vi "quoridor_server.vi"() -> ()   [LabVIEW 2015]
panel:
  in  "STOP":bool
  in  "NON":bool
  in  "OUI":bool
  out "String 6":string
  out "String 5":string
  out "String 4":string
  out "String 3":string
  out "LED1":bool
  out "LED2":bool
  out "LED3":bool
  out "String 2":string
  out "String":string
  out "Play Led":bool
  out "Victoire Client":bool
  out "Victoire Joueur Serveur":bool
  out "?":string
  out "Nombre de murs restants":i32
  out "Timeout":dbl
  out "COMPTEUR LED":dbl
  out "Etat jeu":string
  out "Position joueur":dbl[](array[numeric])
  in  "Bouton gauche (8)":bool
  in  "Bouton droite (4)":bool
  in  "Bouton bas (1)":bool
  in  "Bouton haut (2)":bool
  in  "passer tour":bool
  in  "Haut":bool
  in  "Droite":bool
  in  "X":i32(slide) scale=0.0..8.0
  in  "Y":i32(slide)
  out "Array":u32[][](array[ring])
  # "Règles du jeu : Inspiration Quoridor  \n\nLe but est d’atteindre la ligne d’arrivée à l’autre bout du plateau, rien de plus simple ! \n\nPour cela le joueur peut se déplacer, ou alors poser un mur pour entraver l’adversaire. \n\nLes murs font 2 cases de long, on peut les placer Verticaux ou Horizontaux en sélectionnant la case avec les deux curseurs. \n\nLors des déplacements, un joueur ne peut pas franchir un mur, ni sortir du plateau et encore moins marcher sur l’adversaire ! \n\nEt voilà qui conclut cette explication, bonne chance joueur !"
  # "PS : Ne pas enfermer l’adversaire ni bloquer tous les chemins possibles svp au risque de casser le fun…"
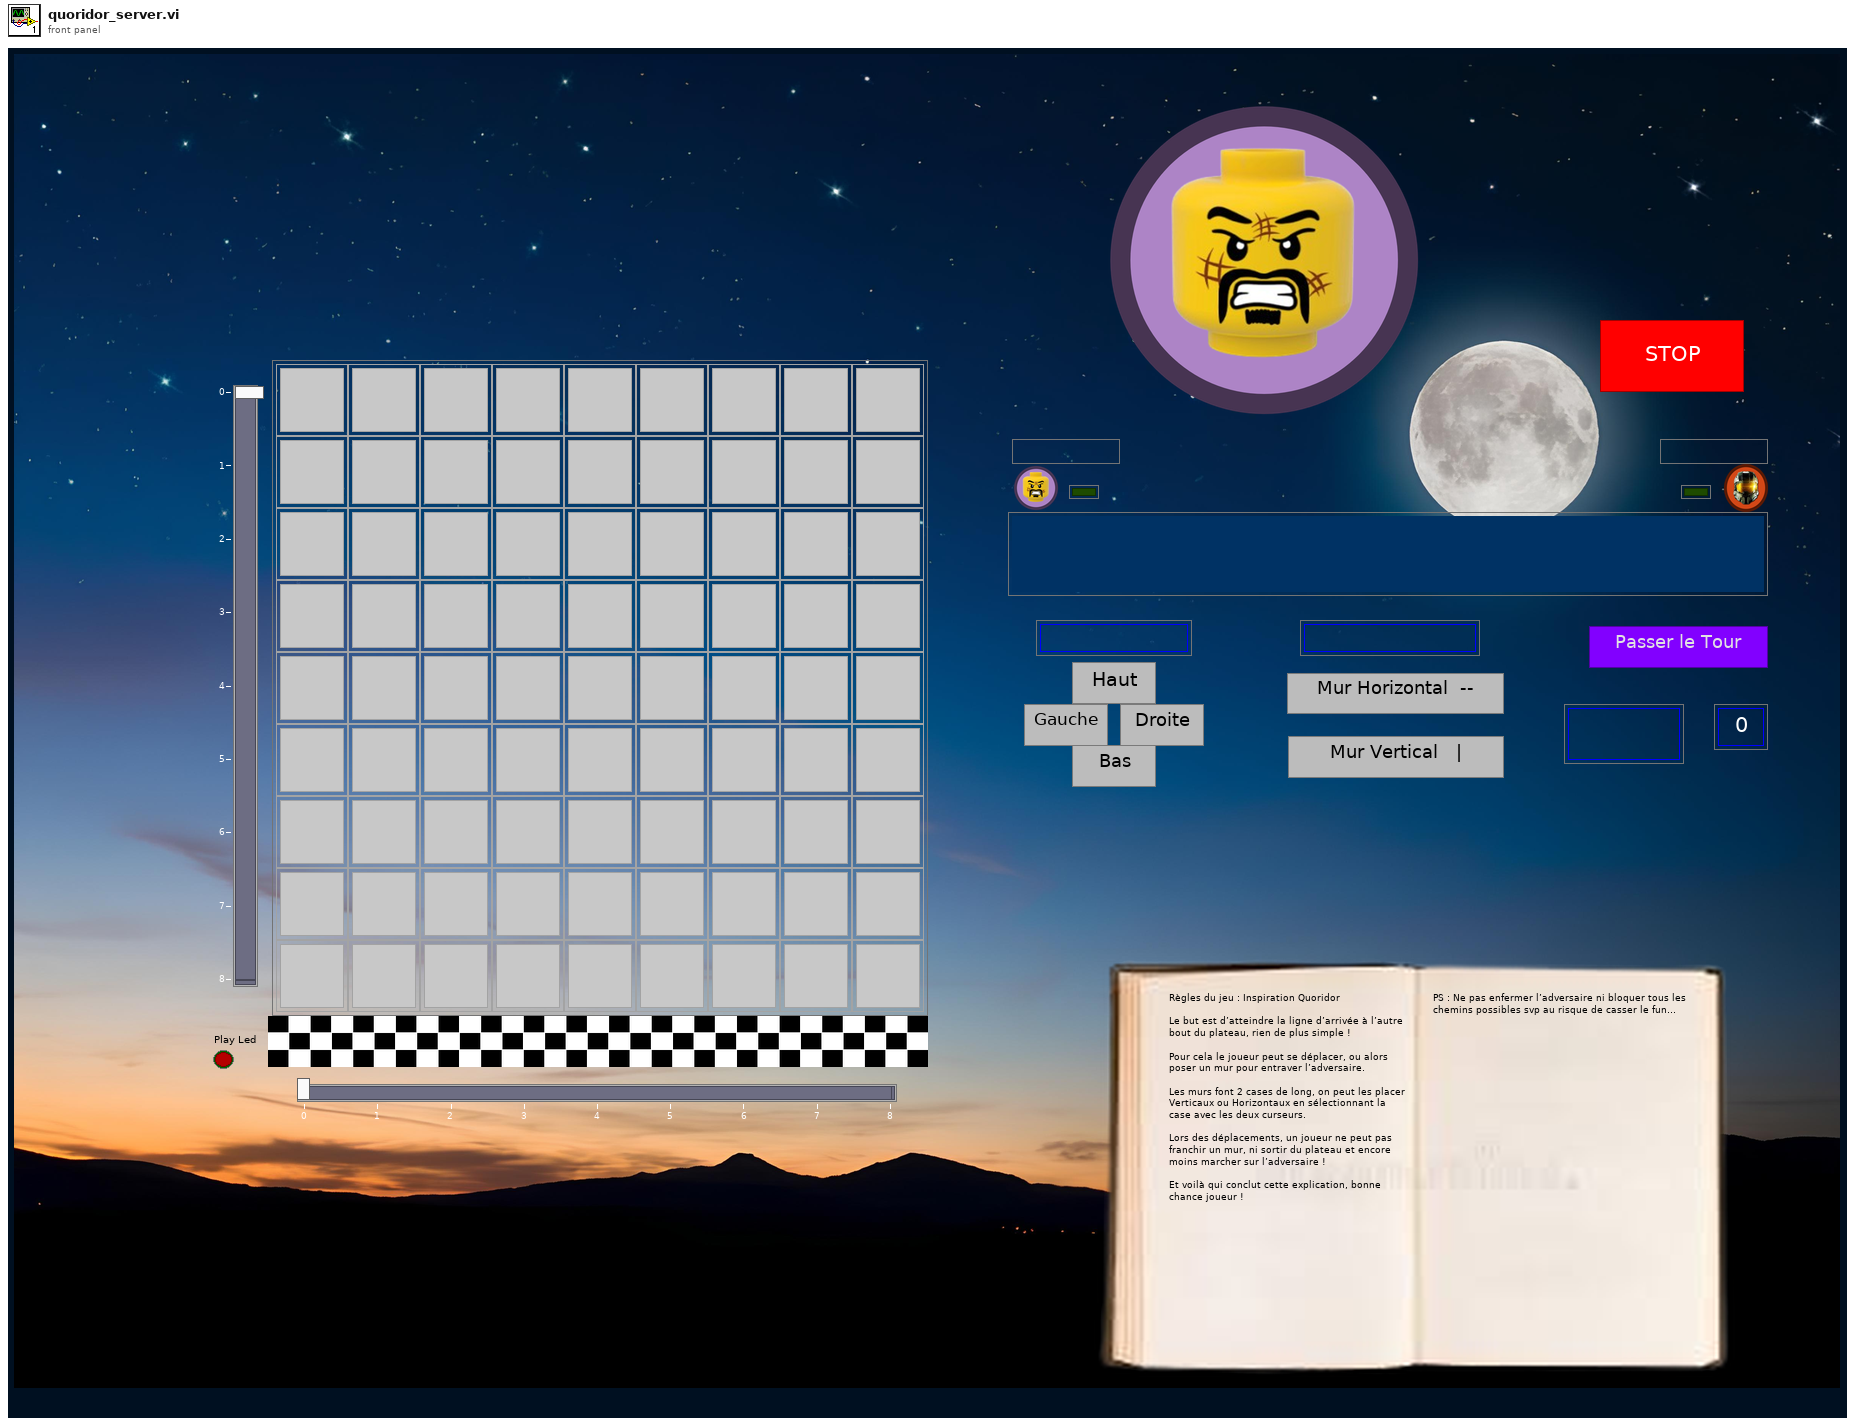
[diagram p1: front panel]
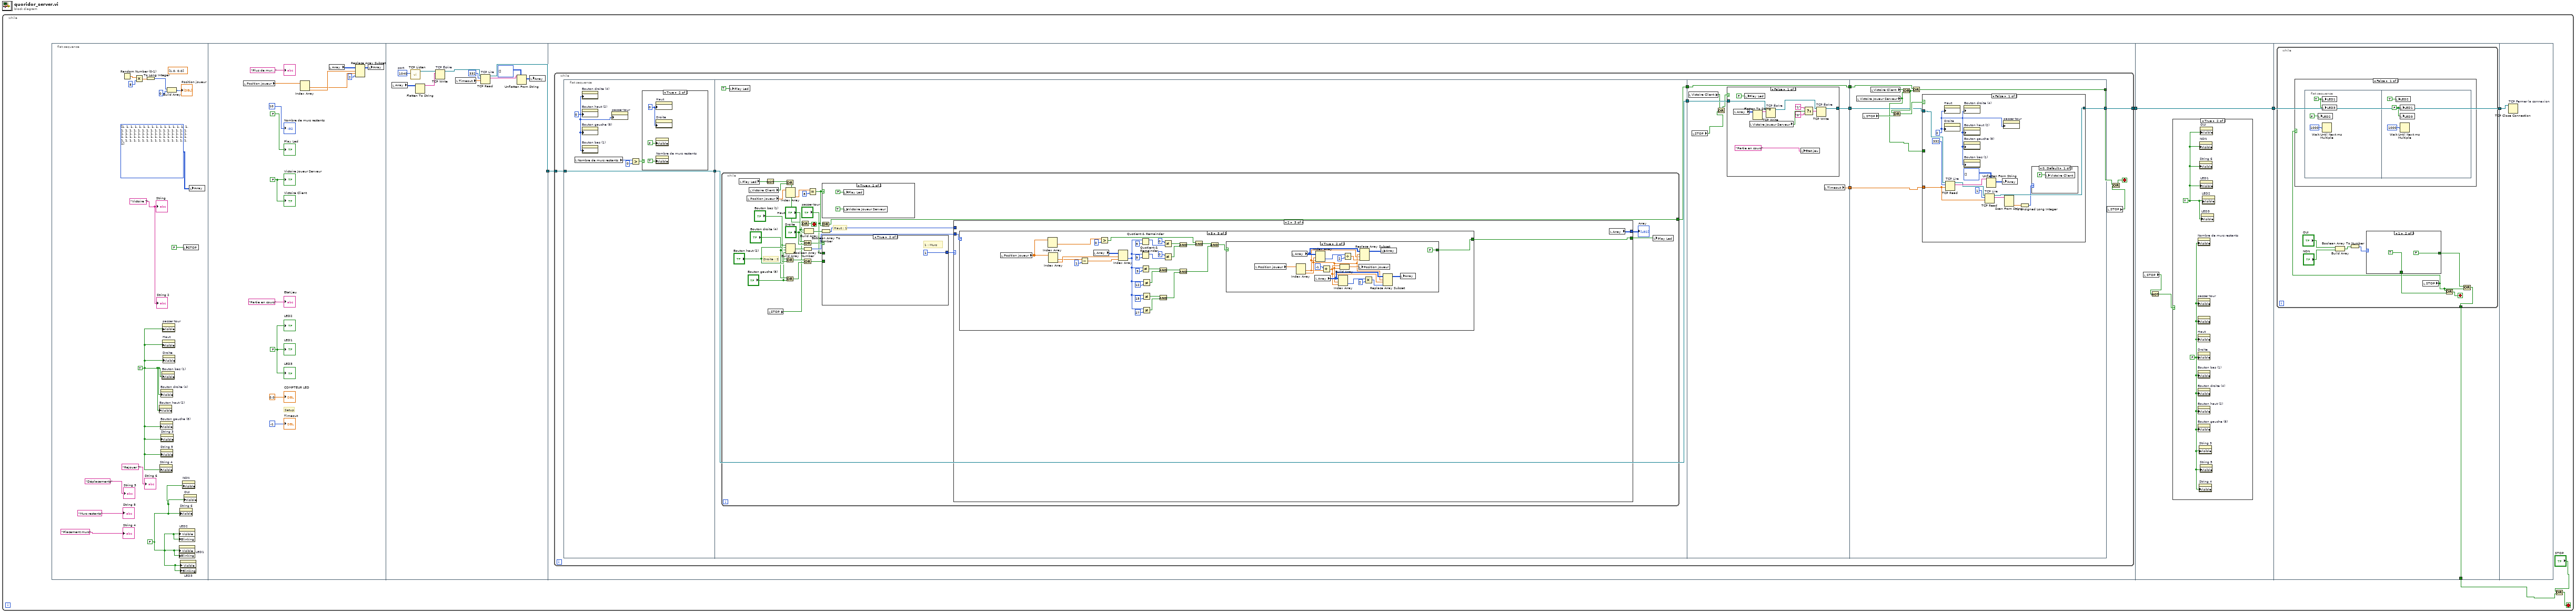
[diagram p0: block diagram]
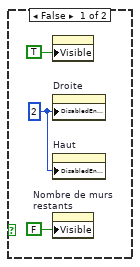
[diagram p2: hidden frame]
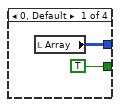
[diagram p4: hidden frame]
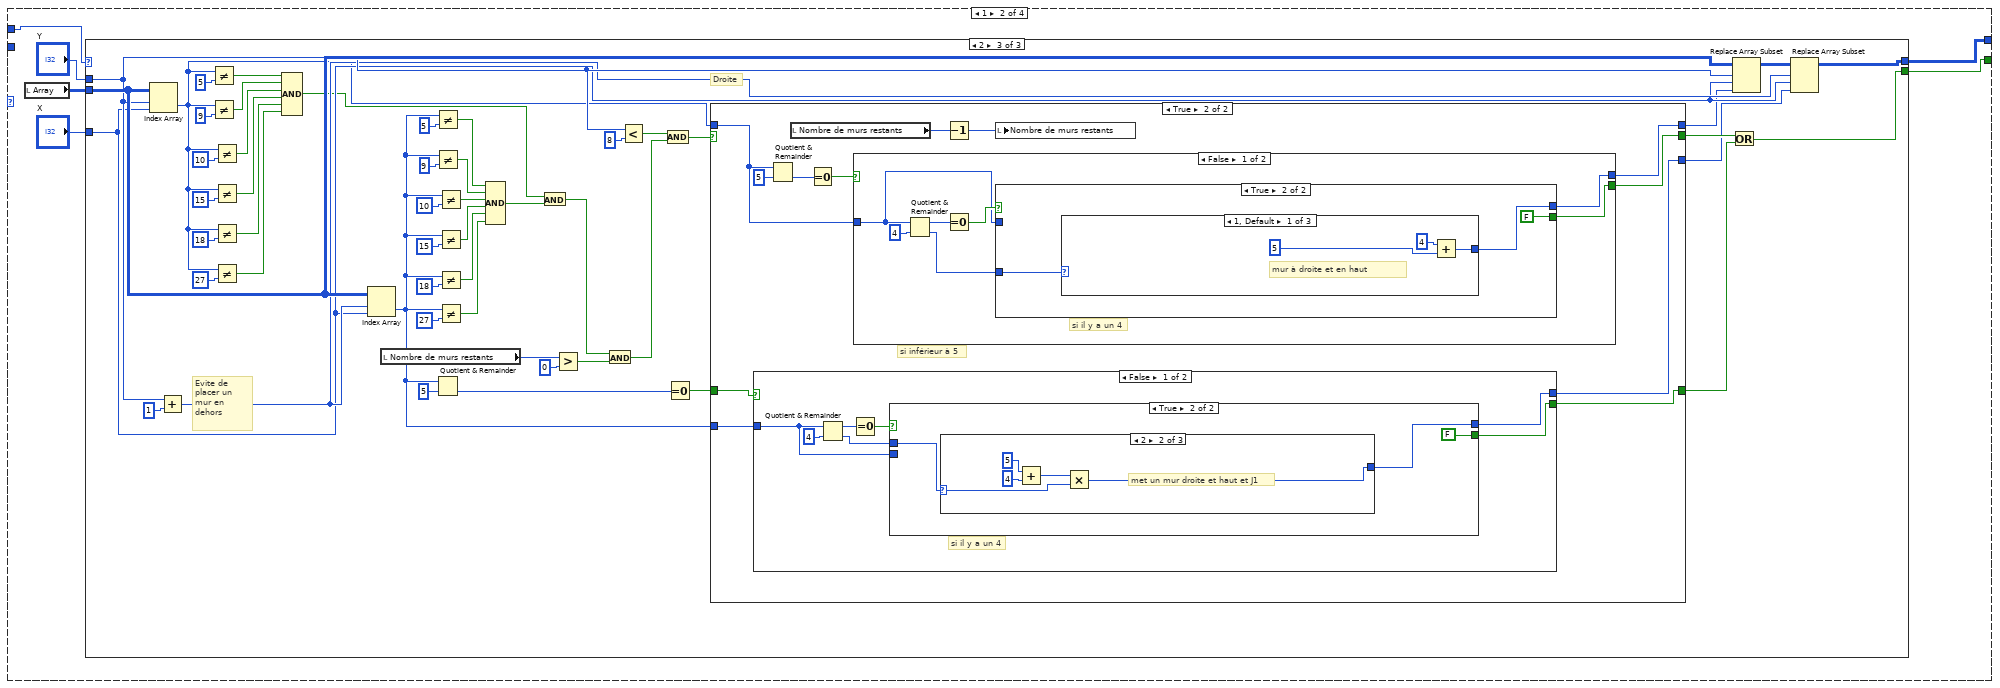
[diagram p5: hidden frame]
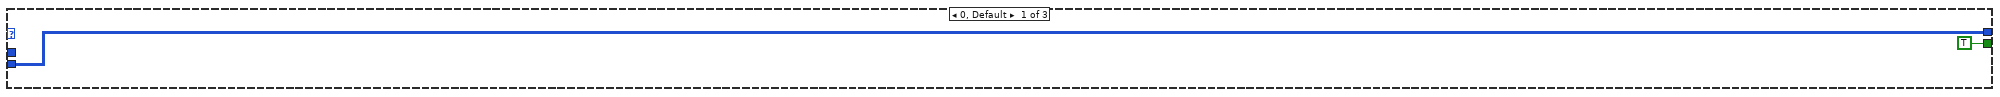
[diagram p6: hidden frame]
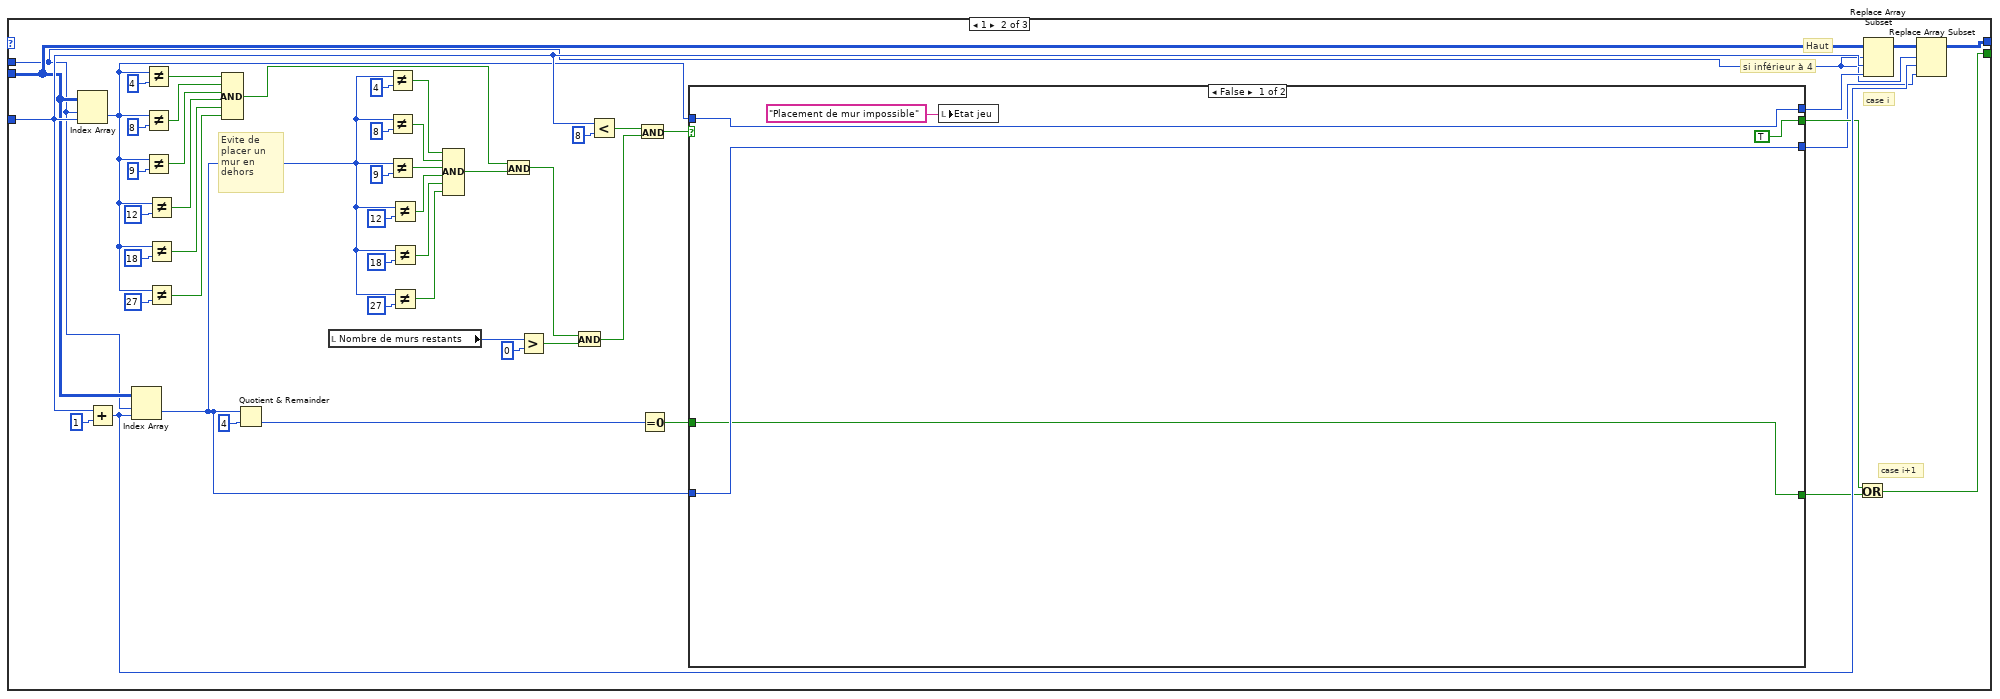
[diagram p7: hidden frame]
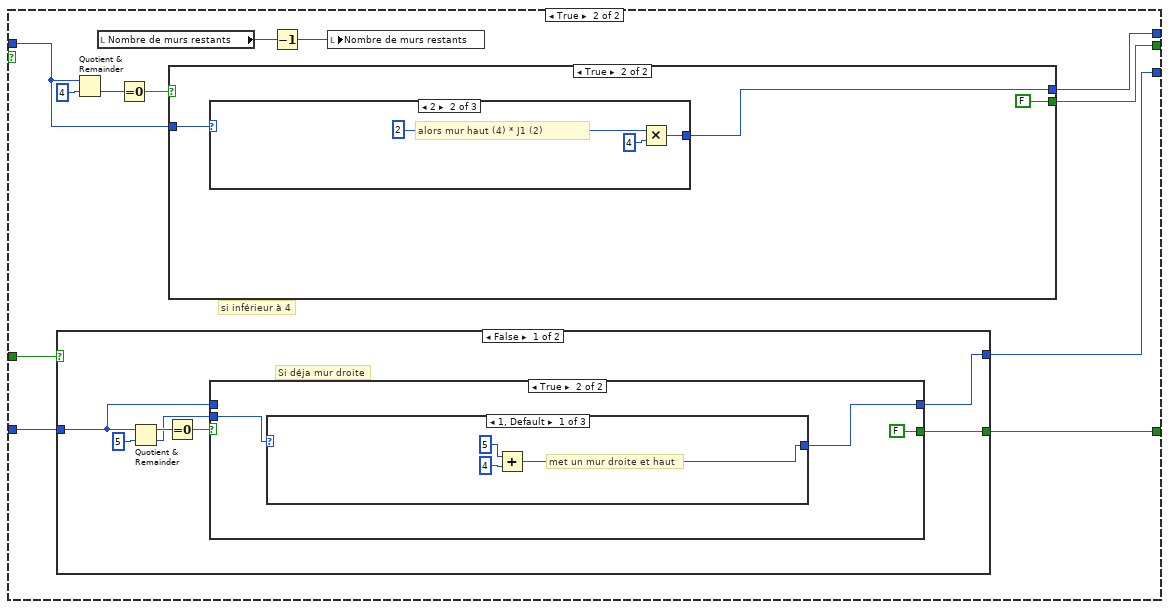
[diagram p8: hidden frame]
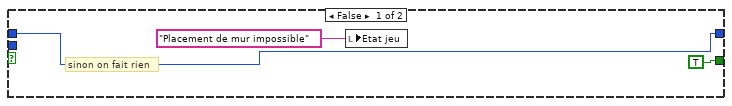
[diagram p9: hidden frame]
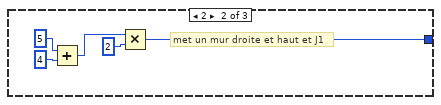
[diagram p10: hidden frame]
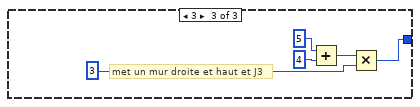
[diagram p11: hidden frame]
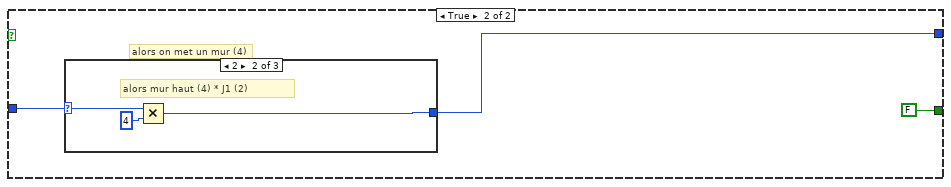
[diagram p12: hidden frame]
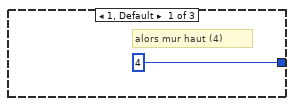
[diagram p13: hidden frame]
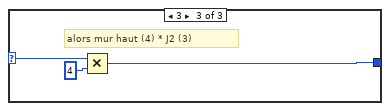
[diagram p14: hidden frame]
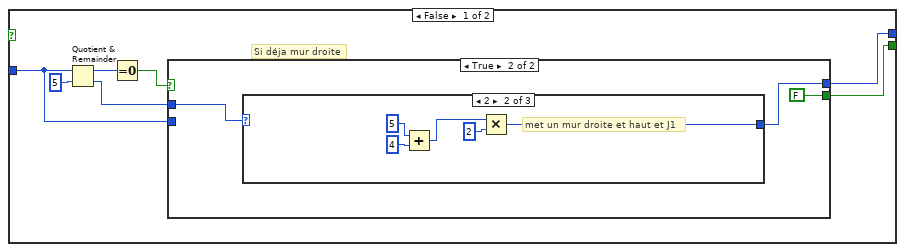
[diagram p15: hidden frame]
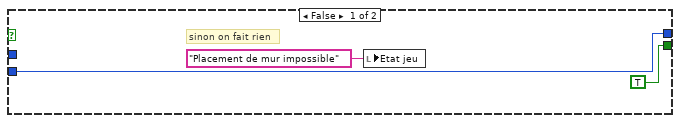
[diagram p16: hidden frame]
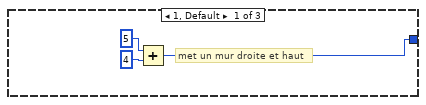
[diagram p17: hidden frame]
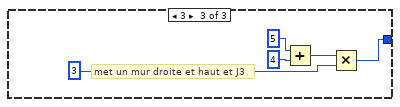
[diagram p18: hidden frame]
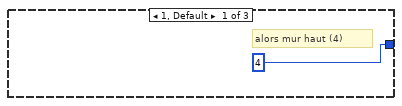
[diagram p19: hidden frame]
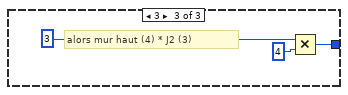
[diagram p20: hidden frame]
diagram:
  n1 = while {
    stop <- w3 stop-if-true
    n2 = flat-sequence {
      tunnel: [w39] -> w7
      tunnel: w7 -> [w48]
      tunnel: [w49] -> w6
      tunnel: w6 -> [w678]
      tunnel: [w678] -> w5
      tunnel: w5 -> [w682]
      tunnel: [w682] -> w4
      tunnel: [w681] -> w1
      tunnel: w4 -> [w703]
      frame #0 {
        w13 = FALSE
        w14 = TRUE
        w15 = "Victoire ?"
        (unwired) dbl[] [1.0, 0.0] ("Position joueur")
        n3 = Random Number (0-1)() -> (number: 0 to 1=w20:dbl)
        n4 = Multiply(x=w20, y=8) -> (x*y=w22:dbl)
        n5 = To Long Integer(number=w22) -> (32bit integer=w17:i32)
        n6 = property on="Bouton haut (2)" class="Bool"("Visible"=w14) -> ()  [unwired: 2 in, 2 out]
        n7 = property on="String 4" class="Str"("Visible"=w14) -> ()  [unwired: 2 in, 2 out]
        n8 = property on="Bouton gauche (8)" class="Bool"("Visible"=w14) -> ()  [unwired: 2 in, 2 out]
        n9 = property on="Bouton droite (4)" class="Bool"("Visible"=w14) -> ()  [unwired: 2 in, 2 out]
        n10 = property on="String 5" class="Str"("Visible"=w14) -> ()  [unwired: 2 in, 2 out]
        n11 = property on="String 3" class="Str"("Visible"=w14) -> ()  [unwired: 2 in, 2 out]
        n12 = property on="Bouton bas (1)" class="Bool"("Visible"=w14) -> ()  [unwired: 2 in, 2 out]
        n13 = property on="passer tour" class="Bool"("Visible"=w14) -> ()  [unwired: 2 in, 2 out]
        n14 = property on="Haut" class="Bool"("Visible"=w14) -> ()  [unwired: 2 in, 2 out]
        n15 = property on="Droite" class="Bool"("Visible"=w14) -> ()  [unwired: 2 in, 2 out]
        n16 = Build Array(w17, 0) -> (→"Position joueur":i32[])
        n17 = property on="LED2" class="Bool (strict)"("Visible"=w13, "Blinking"=w13) -> ()  [unwired: 2 in, 2 out]
        n18 = property on="LED1" class="Bool (strict)"("Visible"=w13, "Blinking"=w13) -> ()  [unwired: 2 in, 2 out]
        n19 = property on="String 6" class="Str"("Visible"=w13) -> ()  [unwired: 2 in, 2 out]
        n20 = property on="LED3" class="Bool (strict)"("Visible"=w13, "Blinking"=w13) -> ()  [unwired: 2 in, 2 out]
        n21 = property on="NON" class="Bool"("Visible"=w13) -> ()  [unwired: 2 in, 2 out]
        n22 = local write "STOP"(FALSE) -> ()
        n23 = property on="OUI" class="Bool"("Visible"=w13) -> ()  [unwired: 2 in, 2 out]
        n24 = local write "Array"(i32[][] [[1, 1, 1, 1, 1, 1, 1, 1, 1], [1, 1, 1, 1, 1, 1, 1, 1, 1], [1, 1, 1, 1, 1, 1, 1, 1, 1], [1, 1, 1, 1, 1, 1, 1, 1, 1], [1, 1, 1, 1, 1, 1, 1, 1, 1], [1, 1, 1, 1, 1, 1, 1, 1, 1], [1, 1, 1, 1, 1, 1, 1, 1, 1], [1, 1, 1, 1, 1, 1, 1, 1, 1], [1, 1, 1, 1, 1, 1, 1, 1, 1]] ("Array 2")) -> ()
        "String" <- w15
        "String 2" <- w15
        "String 3" <- "Déplacements"
        "String 5" <- "Murs restants"
        "String 4" <- "Placement murs"
        "String 6" <- "Rejouer ?"
      }
      frame #1 {
        w23 = FALSE
        w34 = FALSE
        # "Setup"
        n25 = local read "Position joueur"() -> (w32:dbl[])
        n26 = Index Array(array=w32) -> (element #1=w28:dbl, element #2=w29:dbl)  [unwired: 2 in]
        n27 = local read "Array"() -> (w30:u32[][])
        n28 = Replace Array Subset(array=w30, new element=2, index (row)=w29, index (col)=w28) -> (w31:u32[][])
        n29 = local write "Array"(w31) -> ()
        "COMPTEUR LED" <- 0.0
        "Etat jeu" <- "Partie en cours"
        "LED3" <- w34
        "LED1" <- w34
        "LED2" <- w34
        "Timeout" <- -1
        "Play Led" <- FALSE
        "Nombre de murs restants" <- 10
        "?" <- "Plus de mur..."
        "Victoire Joueur Serveur" <- w23
        "Victoire Client" <- w23
      }
      frame #2 {
        w44 = u16 1040  # port
        n30 = local read "Array"() -> (w46:u32[][])
        n31 = call <vilib>:"TCP Listen.vi"("port"=w44) -> ("connection ID"=w47:refnum<k5>)  [unwired: 6 in, 4 out]
        n32 = Flatten To String(anything=w46) -> (data string=w45:string)  [unwired: 3 in, 2 out]
        n33 = TCP Write "TCP Écrire"(connection ID=w47, data in=w45) -> (connection ID out=w40:refnum<k5>)  [unwired: 2 in, 2 out]
        n34 = local read "Timeout"() -> (w38:dbl)
        n35 = TCP Read "TCP Lire"(connection ID=w40, bytes to read=332, 9:w38) -> (connection ID out=w39:refnum<k5>, data out=w42:string)  [unwired: 2 in, 1 out]
        n36 = Unflatten From String(type=i32[][] [], binary string=w42) -> (value=w37:i32[][])  [unwired: 3 in, 2 out]
        n37 = local write "Array"(w37) -> ()
      }
      frame #3 {
        n38 = while {
          tunnel: [w60] -> w49
          tunnel: w48 -> [w58]
          stop <- w51 stop-if-true
          n39 = flat-sequence {
            tunnel: w58 -> [w65]
            tunnel: [w65] -> w54
            tunnel: [w74] -> w57
            tunnel: [w72] -> w55
            tunnel: w54 -> [w74]
            tunnel: [w629] -> w59
            tunnel: w57 -> [w631]
            tunnel: [w630] -> w56
            tunnel: w55 -> [w628]
            tunnel: [w628] -> w53
            tunnel: [w649] -> w60
            tunnel: w59 -> [w646]
            tunnel: w56 -> [w645]
            tunnel: w53 -> [w653]
            tunnel: [w652] -> w52
            frame #0 {
              w61 = 0
              n40 = local read "Nombre de murs restants"() -> (w62:i32)
              n41 = property on="Bouton droite (4)" class="Bool"("DisabledEnum"=w61) -> ()  [unwired: 2 in, 2 out]
              n42 = property on="Bouton haut (2)" class="Bool"("DisabledEnum"=w61) -> ()  [unwired: 2 in, 2 out]
              n43 = property on="Bouton gauche (8)" class="Bool"("DisabledEnum"=w61) -> ()  [unwired: 2 in, 2 out]
              n44 = property on="Bouton bas (1)" class="Bool"("DisabledEnum"=w61) -> ()  [unwired: 2 in, 2 out]
              n45 = property on="passer tour" class="Bool"("DisabledEnum"=w61) -> ()  [unwired: 2 in, 2 out]
              n46 = Greater?(x=w62, y=0) -> (0:w63:bool)
              n47 = case shown="True" w63 {
                frame False {
                  w68 = 2
                  n48 = property class="Str"("Visible"=TRUE) -> ()  [unwired: 2 in, 2 out]
                  n49 = property on="Droite" class="Bool"("DisabledEnum"=w68) -> ()  [unwired: 2 in, 2 out]
                  n50 = property on="Haut" class="Bool"("DisabledEnum"=w68) -> ()  [unwired: 2 in, 2 out]
                  n51 = property on="Nombre de murs restants" class="DigNum (strict)"("Visible"=FALSE) -> ()  [unwired: 2 in, 2 out]
                }
                frame True {
                  w71 = 0
                  n52 = property on="Haut" class="Bool"("DisabledEnum"=w71) -> ()  [unwired: 2 in, 2 out]
                  n53 = property on="Droite" class="Bool"("DisabledEnum"=w71) -> ()  [unwired: 2 in, 2 out]
                  n54 = property class="Str"("Visible"=FALSE) -> ()  [unwired: 2 in, 2 out]
                  n55 = property on="Nombre de murs restants" class="DigNum (strict)"("Visible"=TRUE) -> ()  [unwired: 2 in, 2 out]
                }
              }
            }
            frame #1 {
              n56 = while {
                tunnel: [w78] -> w72
                stop <- w76 stop-if-true
                # "Haut : 1"
                # "Droite : 2"
                n57 = local read "Play Led"() -> (w93:bool)
                n58 = local read "Position joueur"() -> (w81:dbl[])
                n59 = local read "Victoire Client"() -> (w84:bool)
                n60 = Not(x=w93) -> (.not. x?=w85:bool)
                n61 = local read "STOP"() -> (w75:bool)
                n62 = Or(x=w85, y=w84) -> (x .or. y?=w77:bool)
                n63 = Or(x="Bouton haut (2)", y="Bouton bas (1)") -> (x .or. y?=w98:bool)
                n64 = Or(x="Bouton droite (4)", y="Bouton gauche (8)") -> (x .or. y?=w99:bool)
                n65 = Index Array(array=w81) -> (element #2=w82:dbl)  [unwired: 2 in, 1 out]
                n66 = Build Array("Bouton bas (1)", "Bouton haut (2)", "Bouton droite (4)", "Bouton gauche (8)") -> (w100:bool[])
                n67 = Or(x=w77, y=w75) -> (x .or. y?=w76:bool)
                n68 = Or(x="Haut", y="Droite") -> (x .or. y?=w92:bool)
                n69 = Or(x=w98, y=w99) -> (x .or. y?=w91:bool)
                n70 = Boolean Array To Number(Boolean array=w100) -> (number=w88:u32)
                n71 = Build Array("Haut", "Droite") -> (w103:bool[])
                n72 = Equal?(x=w82, y=8) -> (x = y?=w80:bool)
                n73 = Or(x="passer tour", y=w80) -> (x .or. y?=w78:bool)
                n74 = Boolean Array To Number(Boolean array=w103) -> (number=w89:u32)
                n75 = case shown="True" w80 {
                  frame False {
                  }
                  frame True {
                    n76 = local write "Play Led"(FALSE) -> ()
                    n77 = local write "Victoire Joueur Serveur"(TRUE) -> ()
                  }
                }
                n78 = case shown="True" w92 {
                  tunnel: [w618 1] -> w90
                  tunnel: "passer tour" -> [w617 _]
                  tunnel: w91 -> [w616 _]
                  frame False {
                    n79 = case shown="False" w616 {
                      tunnel: [w620 2] -> w618
                      tunnel: w617 -> [w619 _]
                      frame False {
                        n80 = case shown="False" w619 {
                          tunnel: [0 3] -> w620
                          frame False {
                            # "0"
                          }
                          frame True {
                            # "3 : Abandon"
                          }
                        }
                      }
                      frame True {
                        # "2 : Pion"
                      }
                    }
                  }
                  frame True {
                    # "1 : Murs"
                  }
                }
                n81 = case shown="2" w90 {
                  tunnel: w89 -> [_ w112 _ _]
                  tunnel: [w107 w109 w399 w615] -> w86
                  tunnel: w88 -> [_ _ w401 _]
                  tunnel: [TRUE w108 w400 FALSE] -> w87
                  frame 0, Default {
                    n82 = local read "Array"() -> (w107:u32[][])
                  }
                  frame 1 {
                    n83 = local read "Array"() -> (w113:u32[][])
                    n84 = case shown="2" w112 {
                      tunnel: w113 -> [w115 w161 w301]
                      tunnel: "Y" -> [_ w159 w300]
                      tunnel: "X" -> [_ w162 w298]
                      tunnel: [w115 w156 w296] -> w109
                      tunnel: [TRUE w155 w295] -> w108
                      frame 0, Default {
                      }
                      frame 1 {
                        # "si inférieur à 4"
                        # "case i+1"
                        # "case i"
                        # "Evite de placer un mur en dehors"
                        # "Haut"
                        n85 = Index Array(array=w161, index (row)=w159, index (col)=w162) -> (element=w122:u32)
                        n86 = Add(x=w162, y=1) -> (x+y=w160:i32)
                        n87 = Index Array(array=w161, index (row)=w159, index (col)=w160) -> (element=w123:u32)
                        n88 = Not Equal?(x=w122, y=4) -> (x != y?=w144:bool)
                        n89 = Not Equal?(x=w122, y=8) -> (x != y?=w143:bool)
                        n90 = Not Equal?(x=w122, y=9) -> (x != y?=w142:bool)
                        n91 = Not Equal?(x=w122, y=12) -> (x != y?=w141:bool)
                        n92 = Not Equal?(x=w122, y=18) -> (x != y?=w140:bool)
                        n93 = Not Equal?(x=w122, y=27) -> (x != y?=w139:bool)
                        n94 = Compound Arithmetic op=AND(w144, w143, w142, w141, w140, w139) -> (w127:bool)
                        n95 = Quotient & Remainder(x=w123, y=4) -> (floor(x/y)=w157:u32)  [unwired: 1 out]
                        n96 = local read "Nombre de murs restants"() -> (w119:i32)
                        n97 = Not Equal?(x=w123, y=4) -> (x != y?=w133:bool)
                        n98 = Not Equal?(x=w123, y=8) -> (x != y?=w132:bool)
                        n99 = Not Equal?(x=w123, y=9) -> (x != y?=w131:bool)
                        n100 = Not Equal?(x=w123, y=12) -> (x != y?=w130:bool)
                        n101 = Not Equal?(x=w123, y=18) -> (x != y?=w129:bool)
                        n102 = Not Equal?(x=w123, y=27) -> (x != y?=w128:bool)
                        n103 = Compound Arithmetic op=AND(w133, w132, w131, w130, w129, w128) -> (w126:bool)
                        n104 = And(x=w127, y=w126) -> (x .and. y?=w118:bool)
                        n105 = Greater?(x=w119, y=0) -> (0:w116:bool)
                        n106 = And(x=w118, y=w116) -> (x .and. y?=w117:bool)
                        n107 = Less?(x=w162, y=8) -> (x < y?=w124:bool)
                        n108 = And(x=w124, y=w117) -> (x .and. y?=w125:bool)
                        n109 = Equal To 0?(x=w157) -> (x = 0?=w153:bool)
                        n110 = case shown="False" w125 {
                          tunnel: [w171 w180] -> w164
                          tunnel: w122 -> [w171 w179]
                          tunnel: [TRUE w178] -> w154
                          tunnel: w153 -> [w168 w177]
                          tunnel: w123 -> [w169 w176]
                          tunnel: [w168 w175] -> w152
                          tunnel: [w169 w174] -> w151
                          frame False {
                            n111 = local write "Etat jeu"("Placement de mur impossible") -> ()
                          }
                          frame True {
                            # "si inférieur à 4"
                            n112 = case shown="False" w177 {
                              tunnel: [w187 w212] -> w174
                              tunnel: w176 -> [w185 w211]
                              tunnel: [w184 FALSE] -> w175
                              frame False {
                                # "Si déja mur droite"
                                n113 = Quotient & Remainder(x=w185, y=5) -> (x-y*floor(x/y)=w188:u32, floor(x/y)=w186:u32)
                                n114 = Equal To 0?(x=w188) -> (x = 0?=w189:bool)
                                n115 = case shown="True" w189 {
                                tunnel: w186 -> [_ w196]
                                tunnel: [w193 w195] -> w187
                                tunnel: w185 -> [w193 _]
                                tunnel: [TRUE FALSE] -> w184
                                frame False {
                                # "sinon on fait rien"
                                n116 = local write "Etat jeu"("Placement de mur impossible") -> ()
                                }
                                frame True {
                                n117 = case shown="1, Default" w196 {
                                tunnel: [w198 w201 w206] -> w195
                                frame 1, Default {
                                # "met un mur droite et haut"
                                n118 = Add(x=5, y=4) -> (x+y=w198:i32)
                                }
                                frame 2 {
                                # "met un mur droite et haut et J1"
                                n119 = Add(x=5, y=4) -> (x+y=w202:i32)
                                n120 = Multiply(x=w202, y=2) -> (x*y=w201:i32)
                                }
                                frame 3 {
                                # "met un mur droite et haut et J3"
                                n121 = Add(x=5, y=4) -> (x+y=w207:i32)
                                n122 = Multiply(x=w207, y=3) -> (x*y=w206:i32)
                                }
                                }
                                }
                                }
                              }
                              frame True {
                                # "alors on met un mur (4)"
                                n123 = case shown="2" w211 {
                                selector: w211 -> [_ w214 w217]
                                tunnel: [4 w215 w218] -> w212
                                frame 1, Default {
                                # "alors mur haut (4)"
                                }
                                frame 2 {
                                # "alors mur haut (4) * J1 (2)"
                                n124 = Multiply(x=w214, y=4) -> (x*y=w215:u32)
                                }
                                frame 3 {
                                # "alors mur haut (4) * J2 (3)"
                                n125 = Multiply(x=w217, y=4) -> (x*y=w218:u32)
                                }
                                }
                              }
                            }
                            n126 = Quotient & Remainder(x=w179, y=4) -> (floor(x/y)=w182:u32)  [unwired: 1 out]
                            n127 = local read "Nombre de murs restants"() -> (w172:i32)
                            n128 = Equal To 0?(x=w182) -> (x = 0?=w183:bool)
                            n129 = case shown="True" w183 {
                              tunnel: [w223 w247] -> w180
                              tunnel: w179 -> [w221 w248]
                              tunnel: [w220 FALSE] -> w178
                              frame False {
                                # "Si déja mur droite"
                                n130 = Quotient & Remainder(x=w221, y=5) -> (x-y*floor(x/y)=w224:u32, floor(x/y)=w222:u32)
                                n131 = Equal To 0?(x=w224) -> (x = 0?=w225:bool)
                                n132 = case shown="True" w225 {
                                tunnel: w222 -> [_ w232]
                                tunnel: [w228 w231] -> w223
                                tunnel: w221 -> [w228 _]
                                tunnel: [TRUE FALSE] -> w220
                                frame False {
                                # "sinon on fait rien"
                                n133 = local write "Etat jeu"("Placement de mur impossible") -> ()
                                }
                                frame True {
                                n134 = case shown="2" w232 {
                                tunnel: [w233 w236 w241] -> w231
                                frame 1, Default {
                                # "met un mur droite et haut"
                                n135 = Add(x=5, y=4) -> (x+y=w233:i32)
                                }
                                frame 2 {
                                # "met un mur droite et haut et J1"
                                n136 = Add(x=5, y=4) -> (x+y=w238:i32)
                                n137 = Multiply(x=w238, y=2) -> (x*y=w236:i32)
                                }
                                frame 3 {
                                # "met un mur droite et haut et J3"
                                n138 = Add(x=5, y=4) -> (x+y=w243:i32)
                                n139 = Multiply(x=w243, y=3) -> (x*y=w241:i32)
                                }
                                }
                                }
                                }
                              }
                              frame True {
                                n140 = case shown="2" w248 {
                                tunnel: [4 w252 w253] -> w247
                                frame 1, Default {
                                # "alors mur haut (4)"
                                }
                                frame 2 {
                                # "alors mur haut (4) * J1 (2)"
                                n141 = Multiply(x=2, y=4) -> (x*y=w252:i32)
                                }
                                frame 3 {
                                # "alors mur haut (4) * J2 (3)"
                                n142 = Multiply(x=3, y=4) -> (x*y=w253:i32)
                                }
                                }
                              }
                            }
                            n143 = Decrement(x=w172) -> (x-1=w173:i32)
                            n144 = local write "Nombre de murs restants"(w173) -> ()
                          }
                        }
                        n145 = Or(x=w154, y=w152) -> (x .or. y?=w155:bool)
                        n146 = Replace Array Subset(array=w161, new element=w164, index (row)=w159, index (col)=w162) -> (w163:u32[][])
                        n147 = Replace Array Subset(array=w163, new element=w151, index (row)=w159, index (col)=w160) -> (w156:u32[][])
                      }
                      frame 2 {
                        # "Evite de placer un mur en dehors"
                        # "Droite"
                        n148 = Index Array(array=w301, index (row)=w300, index (col)=w298) -> (element=w277:u32)
                        n149 = Add(x=w300, y=1 ("x+y")) -> (x+y=w299:i32)
                        n150 = Not Equal?(x=w277, y=5) -> (x != y?=w284:bool)
                        n151 = Not Equal?(x=w277, y=9) -> (x != y?=w283:bool)
                        n152 = Not Equal?(x=w277, y=10) -> (x != y?=w282:bool)
                        n153 = Not Equal?(x=w277, y=15) -> (x != y?=w281:bool)
                        n154 = Not Equal?(x=w277, y=18) -> (x != y?=w280:bool)
                        n155 = Not Equal?(x=w277, y=27) -> (x != y?=w279:bool)
                        n156 = Compound Arithmetic op=AND(w284, w283, w282, w281, w280, w279) -> (w263:bool)
                        n157 = Index Array(array=w301, index (row)=w299, index (col)=w298) -> (element=w264:u32)
                        n158 = local read "Nombre de murs restants"() -> (w259:i32)
                        n159 = Not Equal?(x=w264, y=5) -> (x != y?=w270:bool)
                        n160 = Not Equal?(x=w264, y=9) -> (x != y?=w269:bool)
                        n161 = Quotient & Remainder(x=w264, y=5) -> (floor(x/y)=w303:u32)  [unwired: 1 out]
                        n162 = Not Equal?(x=w264, y=10) -> (x != y?=w268:bool)
                        n163 = Not Equal?(x=w264, y=15) -> (x != y?=w267:bool)
                        n164 = Not Equal?(x=w264, y=18) -> (x != y?=w266:bool)
                        n165 = Not Equal?(x=w264, y=27) -> (x != y?=w265:bool)
                        n166 = Compound Arithmetic op=AND(w270, w269, w268, w267, w266, w265) -> (w262:bool)
                        n167 = And(x=w263, y=w262) -> (x .and. y?=w258:bool)
                        n168 = Greater?(x=w259, y=0) -> (0:w256:bool)
                        n169 = And(x=w258, y=w256) -> (x .and. y?=w257:bool)
                        n170 = Less?(x=w300, y=8) -> (x < y?=w278:bool)
                        n171 = And(x=w278, y=w257) -> (x .and. y?=w261:bool)
                        n172 = Equal To 0?(x=w303) -> (x = 0?=w291:bool)
                        n173 = case shown="True" w261 {
                          tunnel: w277 -> [w311 w320]
                          tunnel: [w311 w321] -> w297
                          tunnel: [TRUE w318] -> w294
                          tunnel: [w309 w317] -> w293
                          tunnel: [w308 w316] -> w292
                          tunnel: w291 -> [w309 w315]
                          tunnel: w264 -> [w308 w314]
                          frame False {
                            n174 = local write "Etat jeu"("Placement de mur impossible") -> ()
                          }
                          frame True {
                            # "si inférieur à 5"
                            n175 = case shown="False" w315 {
                              tunnel: [w327 w350] -> w316
                              tunnel: [w325 FALSE] -> w317
                              tunnel: w314 -> [w324 w351]
                              frame False {
                                # "si il y a un 4"
                                n176 = Quotient & Remainder(x=w324, y=4) -> (x-y*floor(x/y)=w328:u32, floor(x/y)=w326:u32)
                                n177 = Equal To 0?(x=w328) -> (x = 0?=w329:bool)
                                n178 = case shown="True" w329 {
                                tunnel: w324 -> [w333 _]
                                tunnel: [w333 w335] -> w327
                                tunnel: w326 -> [_ w336]
                                tunnel: [TRUE FALSE] -> w325
                                frame False {
                                # "on ne fait rien"
                                n179 = local write "Etat jeu"("Placement de mur impossible") -> ()
                                }
                                frame True {
                                n180 = case shown="2" w336 {
                                selector: w336 -> [_ w340 w346]
                                tunnel: [w339 w341 w345] -> w335
                                frame 1, Default {
                                # "mur à droite et en haut"
                                n181 = Add(x=4, y=5) -> (x+y=w339:i32)
                                }
                                frame 2 {
                                # "met un mur droite et haut et J1"
                                n182 = Add(x=5, y=4) -> (x+y=w343:i32)
                                n183 = Multiply(x=w343, y=w340) -> (x*y=w341:u32)
                                }
                                frame 3 {
                                # "met un mur droite et haut et J2"
                                n184 = Add(x=5, y=4) -> (x+y=w348:i32)
                                n185 = Multiply(x=w348, y=w346) -> (x*y=w345:u32)
                                }
                                }
                                }
                                }
                              }
                              frame True {
                                n186 = case shown="3" w351 {
                                tunnel: [5 w356 w357] -> w350
                                frame 1, Default {
                                # "alors mur droite (5)"
                                }
                                frame 2 {
                                # "alors mur droite (5) * J1 (2)"
                                n187 = Multiply(x=2, y=5) -> (x*y=w356:i32)
                                }
                                frame 3 {
                                # "alors mur droite (5) * J2 (3)"
                                n188 = Multiply(x=3, y=5) -> (x*y=w357:i32)
                                }
                                }
                              }
                            }
                            n189 = Quotient & Remainder(x=w320, y=5) -> (floor(x/y)=w323:u32)  [unwired: 1 out]
                            n190 = local read "Nombre de murs restants"() -> (w313:i32)
                            n191 = Equal To 0?(x=w323) -> (x = 0?=w319:bool)
                            n192 = case shown="False" w319 {
                              tunnel: [w362 w388] -> w321
                              tunnel: w320 -> [w363 w387]
                              tunnel: [w360 FALSE] -> w318
                              frame False {
                                # "si il y a un 4"
                                n193 = Quotient & Remainder(x=w363, y=4) -> (x-y*floor(x/y)=w364:u32, floor(x/y)=w361:u32)
                                n194 = Equal To 0?(x=w364) -> (x = 0?=w365:bool)
                                n195 = case shown="True" w365 {
                                tunnel: w363 -> [w369 _]
                                tunnel: [w369 w372] -> w362
                                tunnel: w361 -> [_ w371]
                                tunnel: [TRUE FALSE] -> w360
                                frame False {
                                n196 = local write "Etat jeu"("Placement de mur impossible") -> ()
                                }
                                frame True {
                                n197 = case shown="1, Default" w371 {
                                selector: w371 -> [_ w376 w382]
                                tunnel: [w375 w377 w381] -> w372
                                frame 1, Default {
                                # "mur à droite et en haut"
                                n198 = Add(x=4, y=5) -> (x+y=w375:i32)
                                }
                                frame 2 {
                                # "met un mur droite et haut et J1"
                                n199 = Add(x=5, y=4) -> (x+y=w379:i32)
                                n200 = Multiply(x=w379, y=w376) -> (x*y=w377:u32)
                                }
                                frame 3 {
                                # "met un mur droite et haut et J2"
                                n201 = Add(x=5, y=4) -> (x+y=w384:i32)
                                n202 = Multiply(x=w384, y=w382) -> (x*y=w381:u32)
                                }
                                }
                                }
                                }
                              }
                              frame True {
                                n203 = case shown="1, Default" w387 {
                                selector: w387 -> [_ w390 w393 w396]
                                tunnel: [5 w391 w394 w398] -> w388
                                frame 1, Default {
                                # "on met un mur à droite"
                                }
                                frame 2 {
                                # "mur droite + J1"
                                n204 = Multiply(x=5, y=w390) -> (x*y=w391:u32)
                                }
                                frame 3 {
                                # "mur droite +J2"
                                n205 = Multiply(x=5, y=w393) -> (x*y=w394:u32)
                                }
                                frame 4 {
                                # "mur droite + haut"
                                n206 = Add(x=5, y=w396) -> (x+y=w398:u32)
                                }
                                }
                              }
                            }
                            n207 = Decrement(x=w313) -> (x-1=w312:i32)
                            n208 = local write "Nombre de murs restants"(w312) -> ()
                          }
                        }
                        n209 = Or(x=w294, y=w293) -> (x .or. y?=w295:bool)
                        n210 = Replace Array Subset(array=w301, new element=w297, index (row)=w300, index (col)=w298) -> (w304:u32[][])
                        n211 = Replace Array Subset(array=w304, new element=w292, index (row)=w299, index (col)=w298) -> (w296:u32[][])
                      }
                    }
                  }
                  frame 2 {
                    n212 = case shown="8" w401 {
                      tunnel: [TRUE w403 w462 w516 w562] -> w400
                      frame 0, Default {
                      }
                      frame 1 {
                        n213 = local read "Position joueur"() -> (w418:dbl[])
                        n214 = Index Array(array=w418) -> (element #2=w435:dbl)  [unwired: 2 in, 1 out]
                        n215 = Index Array(array=w418) -> (element #1=w432:dbl, element #2=w431:dbl)  [unwired: 2 in]
                        n216 = Add(x=1, y=w431) -> (x+y=w430:dbl)
                        n217 = local read "Array"() -> (w433:u32[][])
                        n218 = Less?(x=w435, y=8) -> (x < y?=w425:bool)
                        n219 = Index Array(array=w433, index (row)=w430, index (col)=w432) -> (element=w405:u32)
                        n220 = Quotient & Remainder(x=w405, y=4) -> (x-y*floor(x/y)=w427:u32)  [unwired: 1 out]
                        n221 = Quotient & Remainder(x=w405, y=9) -> (x-y*floor(x/y)=w423:u32)  [unwired: 1 out]
                        n222 = Not Equal?(x=w405, y=3) -> (x != y?=w414:bool)
                        n223 = Not Equal?(x=w405, y=12) -> (x != y?=w413:bool)
                        n224 = Not Equal?(x=w405, y=15) -> (x != y?=w409:bool)
                        n225 = Not Equal?(x=w405, y=27) -> (x != y?=w410:bool)
                        n226 = And(x=w414, y=w413) -> (x .and. y?=w412:bool)
                        n227 = And(x=w409, y=w410) -> (x .and. y?=w411:bool)
                        n228 = Not Equal?(x=0, y=w427) -> (x != y?=w420:bool)
                        n229 = Not Equal?(x=0, y=w423) -> (x != y?=w419:bool)
                        n230 = And(x=w420, y=w419) -> (x .and. y?=w421:bool)
                        n231 = And(x=w412, y=w411) -> (x .and. y?=w408:bool)
                        n232 = And(x=w425, y=w421) -> (x .and. y?=w407:bool)
                        n233 = And(x=w407, y=w408) -> (x .and. y?=w406:bool)
                        n234 = case shown="True" w406 {
                          tunnel: [TRUE FALSE] -> w403
                          frame False {
                            n235 = local write "Etat jeu"("Déplacement impossible") -> ()
                          }
                          frame True {
                            n236 = local read "Position joueur"() -> (w452:dbl[])
                            n237 = local read "Array"() -> (w449:u32[][])
                            n238 = Index Array(array=w452) -> (element #1=w439:dbl, element #2=w448:dbl)  [unwired: 2 in]
                            n239 = local read "Array"() -> (w441:u32[][])
                            n240 = Index Array(array=w449, index (row)=w448, index (col)=w439) -> (element=w446:u32)
                            n241 = Add(x=w448, y=1) -> (x+y=w440:dbl)
                            n242 = Index Array(array=w441, index (row)=w440, index (col)=w439) -> (element=w442:u32)
                            n243 = Build Array(w439, w440) -> (w451:dbl[])
                            n244 = Divide(x=w446, y=2) -> (x/y=w445:dbl)
                            n245 = local write "Position joueur"(w451) -> ()
                            n246 = Replace Array Subset(array=w449, new element=w445, index (row)=w448, index (col)=w439) -> (w453:u32[][])
                            n247 = Multiply(x=w442, y=2) -> (x*y=w444:u32)
                            n248 = local write "Array"(w453) -> ()
                            n249 = Replace Array Subset(array=w441, new element=w444, index (row)=w440, index (col)=w439) -> (w450:u32[][])
                            n250 = local write "Array"(w450) -> ()
                          }
                        }
                      }
                      frame 2 {
                        n251 = local read "Position joueur"() -> (w486:dbl[])
                        n252 = Index Array(array=w486) -> (element #1=w458:dbl, element #2=w457:dbl)  [unwired: 2 in]
                        n253 = local read "Array"() -> (w455:u32[][])
                        n254 = Subtract(x=w457, y=1) -> (x-y=w459:dbl)
                        n255 = Index Array(array=w455, index (row)=w457, index (col)=w458) -> (element=w456:u32)
                        n256 = Index Array(array=w455, index (row)=w459, index (col)=w458) -> (element=w461:u32)
                        n257 = local read "Position joueur"() -> (w487:dbl[])
                        n258 = Quotient & Remainder(x=w456, y=4) -> (x-y*floor(x/y)=w482:u32)  [unwired: 1 out]
                        n259 = Quotient & Remainder(x=w456, y=9) -> (x-y*floor(x/y)=w480:u32)  [unwired: 1 out]
                        n260 = Not Equal?(x=w461, y=3) -> (x != y?=w472:bool)
                        n261 = Not Equal?(x=w461, y=12) -> (x != y?=w471:bool)
                        n262 = Not Equal?(x=w461, y=15) -> (x != y?=w467:bool)
                        n263 = Not Equal?(x=w461, y=27) -> (x != y?=w468:bool)
                        n264 = And(x=w472, y=w471) -> (x .and. y?=w470:bool)
                        n265 = And(x=w467, y=w468) -> (x .and. y?=w469:bool)
                        n266 = Index Array(array=w487) -> (element #2=w488:dbl)  [unwired: 2 in, 1 out]
                        n267 = Not Equal?(x=0, y=w482) -> (x != y?=w477:bool)
                        n268 = Not Equal?(x=0, y=w480) -> (x != y?=w478:bool)
                        n269 = And(x=w477, y=w478) -> (x .and. y?=w476:bool)
                        n270 = And(x=w470, y=w469) -> (x .and. y?=w465:bool)
                        n271 = Greater?(x=w488, y=0) -> (0:w484:bool)
                        n272 = And(x=w484, y=w476) -> (x .and. y?=w466:bool)
                        n273 = And(x=w466, y=w465) -> (x .and. y?=w464:bool)
                        n274 = case shown="True" w464 {
                          tunnel: [TRUE FALSE] -> w462
                          frame False {
                            n275 = local write "Etat jeu"("Déplacement impossible") -> ()
                          }
                          frame True {
                            n276 = local read "Position joueur"() -> (w506:dbl[])
                            n277 = local read "Array"() -> (w502:u32[][])
                            n278 = Index Array(array=w506) -> (element #1=w494:dbl, element #2=w503:dbl)  [unwired: 2 in]
                            n279 = local read "Array"() -> (w496:u32[][])
                            n280 = Index Array(array=w502, index (row)=w503, index (col)=w494) -> (element=w498:u32)
                            n281 = Add(x=w503, y=-1) -> (x+y=w495:dbl)
                            n282 = Index Array(array=w496, index (row)=w495, index (col)=w494) -> (element=w493:u32)
                            n283 = Build Array(w494, w495) -> (w505:dbl[])
                            n284 = Divide(x=w498, y=2) -> (x/y=w501:dbl)
                            n285 = local write "Position joueur"(w505) -> ()
                            n286 = Replace Array Subset(array=w502, new element=w501, index (row)=w503, index (col)=w494) -> (w507:u32[][])
                            n287 = Multiply(x=w493, y=2) -> (x*y=w497:u32)
                            n288 = local write "Array"(w507) -> ()
                            n289 = Replace Array Subset(array=w496, new element=w497, index (row)=w495, index (col)=w494) -> (w504:u32[][])
                            n290 = local write "Array"(w504) -> ()
                          }
                        }
                      }
                      frame 4 {
                        n291 = local read "Position joueur"() -> (w530:dbl[])
                        n292 = local read "Array"() -> (w511:u32[][])
                        n293 = Index Array(array=w530) -> (element #1=w542:dbl)  [unwired: 2 in, 1 out]
                        n294 = Index Array(array=w530) -> (element #1=w509:dbl, element #2=w510:dbl)  [unwired: 2 in]
                        n295 = Index Array(array=w511, index (row)=w510, index (col)=w509) -> (element=w512:u32)
                        n296 = Add(x=w509, y=1) -> (x+y=w513:dbl)
                        n297 = Index Array(array=w511, index (row)=w510, index (col)=w513) -> (element=w515:u32)
                        n298 = Quotient & Remainder(x=w512, y=5) -> (x-y*floor(x/y)=w539:u32)  [unwired: 1 out]
                        n299 = Quotient & Remainder(x=w512, y=9) -> (x-y*floor(x/y)=w536:u32)  [unwired: 1 out]
                        n300 = Not Equal?(x=0, y=w539) -> (x != y?=w533:bool)
                        n301 = Not Equal?(x=0, y=w536) -> (x != y?=w532:bool)
                        n302 = Not Equal?(x=w515, y=3) -> (x != y?=w525:bool)
                        n303 = Not Equal?(x=w515, y=12) -> (x != y?=w524:bool)
                        n304 = Not Equal?(x=w515, y=15) -> (x != y?=w520:bool)
                        n305 = Not Equal?(x=w515, y=27) -> (x != y?=w521:bool)
                        n306 = And(x=w533, y=w532) -> (x .and. y?=w534:bool)
                        n307 = And(x=w525, y=w524) -> (x .and. y?=w523:bool)
                        n308 = And(x=w520, y=w521) -> (x .and. y?=w522:bool)
                        n309 = Less?(x=w542, y=8) -> (x < y?=w531:bool)
                        n310 = And(x=w531, y=w534) -> (x .and. y?=w519:bool)
                        n311 = And(x=w523, y=w522) -> (x .and. y?=w518:bool)
                        n312 = And(x=w519, y=w518) -> (x .and. y?=w517:bool)
                        n313 = case shown="True" w517 {
                          tunnel: [TRUE FALSE] -> w516
                          frame False {
                            n314 = local write "Etat jeu"("Déplacement impossible") -> ()
                          }
                          frame True {
                            n315 = local read "Position joueur"() -> (w561:dbl[])
                            n316 = local read "Array"() -> (w551:u32[][])
                            n317 = Index Array(array=w561) -> (element #1=w547:dbl, element #2=w548:dbl)  [unwired: 2 in]
                            n318 = local read "Array"() -> (w550:u32[][])
                            n319 = Index Array(array=w551, index (row)=w548, index (col)=w547) -> (element=w554:u32)
                            n320 = Add(x=1, y=w547) -> (x+y=w549:dbl)
                            n321 = Index Array(array=w550, index (row)=w548, index (col)=w549) -> (element=w556:u32)
                            n322 = Build Array(w549, w548) -> (w558:dbl[])
                            n323 = Divide(x=w554, y=2) -> (x/y=w553:dbl)
                            n324 = local write "Position joueur"(w558) -> ()
                            n325 = Replace Array Subset(array=w551, new element=w553, index (row)=w548, index (col)=w547) -> (w560:u32[][])
                            n326 = Multiply(x=w556, y=2) -> (x*y=w552:u32)
                            n327 = local write "Array"(w560) -> ()
                            n328 = Replace Array Subset(array=w550, new element=w552, index (row)=w548, index (col)=w549) -> (w557:u32[][])
                            n329 = local write "Array"(w557) -> ()
                          }
                        }
                      }
                      frame 8 {
                        n330 = local read "Position joueur"() -> (w585:dbl[])
                        n331 = Index Array(array=w585) -> (element #1=w577:dbl)  [unwired: 2 in, 1 out]
                        n332 = Index Array(array=w585) -> (element #1=w579:dbl, element #2=w581:dbl)  [unwired: 2 in]
                        n333 = Subtract(x=w579, y=1) -> (x-y=w580:dbl)
                        n334 = local read "Array"() -> (w584:u32[][])
                        n335 = Greater?(x=w577, y=0) -> (0:w582:bool)
                        n336 = Index Array(array=w584, index (row)=w581, index (col)=w580) -> (element=w565:u32)
                        n337 = Quotient & Remainder(x=w565, y=5) -> (x-y*floor(x/y)=w593:u32)  [unwired: 1 out]
                        n338 = Quotient & Remainder(x=w565, y=9) -> (x-y*floor(x/y)=w590:u32)  [unwired: 1 out]
                        n339 = Not Equal?(x=w565, y=3) -> (x != y?=w572:bool)
                        n340 = Not Equal?(x=w565, y=12) -> (x != y?=w571:bool)
                        n341 = Not Equal?(x=w565, y=15) -> (x != y?=w563:bool)
                        n342 = Not Equal?(x=w565, y=27) -> (x != y?=w564:bool)
                        n343 = And(x=w572, y=w571) -> (x .and. y?=w570:bool)
                        n344 = And(x=w563, y=w564) -> (x .and. y?=w569:bool)
                        n345 = Not Equal?(x=0, y=w593) -> (x != y?=w587:bool)
                        n346 = Not Equal?(x=0, y=w590) -> (x != y?=w586:bool)
                        n347 = And(x=w587, y=w586) -> (x .and. y?=w588:bool)
                        n348 = And(x=w570, y=w569) -> (x .and. y?=w568:bool)
                        n349 = And(x=w582, y=w588) -> (x .and. y?=w567:bool)
                        n350 = And(x=w567, y=w568) -> (x .and. y?=w566:bool)
                        n351 = case shown="True" w566 {
                          tunnel: [TRUE FALSE] -> w562
                          frame False {
                            n352 = local write "Etat jeu"("Déplacement impossible") -> ()
                          }
                          frame True {
                            n353 = local read "Position joueur"() -> (w613:dbl[])
                            n354 = local read "Array"() -> (w604:u32[][])
                            n355 = Index Array(array=w613) -> (element #1=w598:dbl, element #2=w599:dbl)  [unwired: 2 in]
                            n356 = local read "Array"() -> (w603:u32[][])
                            n357 = Index Array(array=w604, index (row)=w599, index (col)=w598) -> (element=w606:u32)
                            n358 = Add(x=-1, y=w598) -> (x+y=w601:dbl)
                            n359 = Index Array(array=w603, index (row)=w599, index (col)=w601) -> (element=w608:u32)
                            n360 = Build Array(w601, w599) -> (w610:dbl[])
                            n361 = Divide(x=w606, y=2) -> (x/y=w600:dbl)
                            n362 = local write "Position joueur"(w610) -> ()
                            n363 = Replace Array Subset(array=w604, new element=w600, index (row)=w599, index (col)=w598) -> (w612:u32[][])
                            n364 = Multiply(x=w608, y=2) -> (x*y=w602:u32)
                            n365 = local write "Array"(w612) -> ()
                            n366 = Replace Array Subset(array=w603, new element=w602, index (row)=w599, index (col)=w601) -> (w609:u32[][])
                            n367 = local write "Array"(w609) -> ()
                          }
                        }
                      }
                    }
                    n368 = local read "Array"() -> (w399:u32[][])
                  }
                  frame 3 {
                    n369 = local read "Array"() -> (w615:u32[][])
                  }
                }
                "Array" <- w86
                n370 = local write "Play Led"(w87) -> ()
              }
              n371 = local write "Play Led"(TRUE) -> ()
            }
            frame #2 {
              n372 = local read "Victoire Client"() -> (w627:bool)
              n373 = local read "STOP"() -> (w625:bool)
              n374 = Or(x=w627, y=w625) -> (x .or. y?=w626:bool)
              n375 = case shown="False" w626 {
                tunnel: w631 -> [w640 w644]
                tunnel: [w636 w644] -> w629
                frame False {
                  n376 = local read "Array"() -> (w642:u32[][])
                  n377 = local write "Play Led"(FALSE) -> ()
                  n378 = local read "Victoire Joueur Serveur"() -> (w633:bool)
                  n379 = Flatten To String(anything=w642) -> (data string=w641:string)  [unwired: 3 in, 2 out]
                  n380 = TCP Write "TCP Écrire"(connection ID=w640, data in=w641) -> (connection ID out=w635:refnum<k5>)  [unwired: 2 in, 2 out]
                  n381 = local write "Etat jeu"("Partie en cours") -> ()
                  n382 = Select(t="1", s=w633, f="0") -> (s? t:f=w634:string)
                  n383 = TCP Write "TCP Écrire"(connection ID=w635, data in=w634) -> (connection ID out=w636:refnum<k5>)  [unwired: 2 in, 2 out]
                }
                frame True {
                  n384 = local write "Play Led"(FALSE) -> ()
                }
              }
              n385 = local read "Timeout"() -> (w630:dbl)
            }
            frame #3 {
              n386 = local read "Victoire Joueur Serveur"() -> (w648:bool)
              n387 = local read "STOP"() -> (w650:bool)
              n388 = local read "Victoire Client"() -> (w654:bool)
              n389 = Or(x=w654, y=w648) -> (x .or. y?=w651:bool)
              n390 = Or(x=w651, y=w650) -> (x .or. y?=w647:bool)
              n391 = Or(x=w653, y=w651) -> (x .or. y?=w652:bool)
              n392 = case shown="False" w647 {
                tunnel: [w661 w670] -> w649
                tunnel: w645 -> [w658 _]
                tunnel: w648 -> [_ w671]
                tunnel: w646 -> [w655 w670]
                frame False {
                  w656 = 2
                  n393 = property on="Haut" class="Bool"("DisabledEnum"=w656) -> ()  [unwired: 2 in, 2 out]
                  n394 = property on="Droite" class="Bool"("DisabledEnum"=w656) -> ()  [unwired: 2 in, 2 out]
                  n395 = TCP Read "TCP Lire"(connection ID=w655, bytes to read=332, 9:w658) -> (connection ID out=w660:refnum<k5>, data out=w666:string)  [unwired: 2 in, 1 out]
                  n396 = property on="Bouton droite (4)" class="Bool"("DisabledEnum"=w656) -> ()  [unwired: 2 in, 2 out]
                  n397 = property on="Bouton haut (2)" class="Bool"("DisabledEnum"=w656) -> ()  [unwired: 2 in, 2 out]
                  n398 = property on="Bouton gauche (8)" class="Bool"("DisabledEnum"=w656) -> ()  [unwired: 2 in, 2 out]
                  n399 = property on="Bouton bas (1)" class="Bool"("DisabledEnum"=w656) -> ()  [unwired: 2 in, 2 out]
                  n400 = TCP Read "TCP Lire"(connection ID=w660, bytes to read=1, 9:w658) -> (connection ID out=w661:refnum<k5>, data out=w663:string)  [unwired: 2 in, 1 out]
                  n401 = Unflatten From String(type=i32[][] [], binary string=w666) -> (value=w665:i32[][])  [unwired: 3 in, 2 out]
                  n402 = local write "Array"(w665) -> ()
                  n403 = property on="passer tour" class="Bool"("DisabledEnum"=w656) -> ()  [unwired: 2 in, 2 out]
                  n404 = Scan From String(input string=w663) -> (output 1=w662:dbl)  [unwired: 4 in, 3 out]
                  n405 = To Unsigned Long Integer(number=w662) -> (unsigned 32bit integer=w659:u32)
                  n406 = case shown="0, Default" w659 {
                    frame 0, Default {
                      n407 = local write "Victoire Client"(FALSE) -> ()
                    }
                    frame 1 {
                      n408 = local write "Victoire Client"(TRUE) -> ()
                    }
                  }
                }
                frame True {
                  n409 = case shown="True" w671 {
                    frame False {
                      w672 = cluster{u32, u32}[] [{16711680, 16711680}, {16744448, 16744448}] ("Colors [4]")
                      n410 = local write "Etat jeu"("Défaite...") -> ()
                      n411 = property on="LED1" class="Bool (strict)"("Colors [4]"=w672) -> ()  [unwired: 2 in, 2 out]
                      n412 = property on="LED3" class="Bool (strict)"("Colors [4]"=w672) -> ()  [unwired: 2 in, 2 out]
                      n413 = property on="LED2" class="Bool (strict)"("Colors [4]"=w672) -> ()  [unwired: 2 in, 2 out]
                    }
                    frame True {
                      w674 = cluster{u32, u32}[] [{65280, 65280}, {255, 255}, {49647, 1245154}, {0, 0}, {16777215, 16711422}, {16738816, 15690752}] ("Colors [4]")
                      n414 = property on="LED1" class="Bool (strict)"("Colors [4]"=w674) -> ()  [unwired: 2 in, 2 out]
                      n415 = property on="LED2" class="Bool (strict)"("Colors [4]"=w674) -> ()  [unwired: 2 in, 2 out]
                      n416 = property on="LED3" class="Bool (strict)"("Colors [4]"=w674) -> ()  [unwired: 2 in, 2 out]
                      n417 = local write "Etat jeu"("Victoire Brickambolesque !") -> ()
                    }
                  }
                }
              }
            }
          }
          n418 = local read "STOP"() -> (w50:bool)
          n419 = Or(x=w52, y=w50) -> (x .or. y?=w51:bool)
        }
      }
      frame #4 {
        n420 = local read "STOP"() -> (w677:bool)
        n421 = Not(x=w677) -> (.not. x?=w676:bool)
        n422 = case shown="True" w676 {
          frame False {
          }
          frame True {
            w679 = TRUE
            w680 = FALSE
            n423 = property on="Nombre de murs restants" class="DigNum (strict)"("Visible"=w680) -> ()  [unwired: 2 in, 2 out]
            n424 = property on="passer tour" class="Bool"("Visible"=w680) -> ()  [unwired: 2 in, 2 out]
            n425 = property class="Str"("Visible"=w680) -> ()  [unwired: 2 in, 2 out]
            n426 = property on="Haut" class="Bool"("Visible"=w680) -> ()  [unwired: 2 in, 2 out]
            n427 = property on="Droite" class="Bool"("Visible"=w680) -> ()  [unwired: 2 in, 2 out]
            n428 = property on="Bouton bas (1)" class="Bool"("Visible"=w680) -> ()  [unwired: 2 in, 2 out]
            n429 = property on="Bouton droite (4)" class="Bool"("Visible"=w680) -> ()  [unwired: 2 in, 2 out]
            n430 = property on="Bouton haut (2)" class="Bool"("Visible"=w680) -> ()  [unwired: 2 in, 2 out]
            n431 = property on="Bouton gauche (8)" class="Bool"("Visible"=w680) -> ()  [unwired: 2 in, 2 out]
            n432 = property on="String 3" class="Str"("Visible"=w680) -> ()  [unwired: 2 in, 2 out]
            n433 = property on="String 4" class="Str"("Visible"=w680) -> ()  [unwired: 2 in, 2 out]
            n434 = property on="NON" class="Bool"("Visible"=w679) -> ()  [unwired: 2 in, 2 out]
            n435 = property on="String 6" class="Str"("Visible"=w679) -> ()  [unwired: 2 in, 2 out]
            n436 = property on="String 5" class="Str"("Visible"=w680) -> ()  [unwired: 2 in, 2 out]
            n437 = property on="OUI" class="Bool"("Visible"=w679) -> ()  [unwired: 2 in, 2 out]
            n438 = property on="LED1" class="Bool (strict)"("Visible"=w679) -> ()  [unwired: 2 in, 2 out]
            n439 = property on="LED3" class="Bool (strict)"("Visible"=w679) -> ()  [unwired: 2 in, 2 out]
            n440 = property on="LED2" class="Bool (strict)"("Visible"=w679) -> ()  [unwired: 2 in, 2 out]
          }
        }
      }
      frame #5 {
        n441 = while {
          tunnel: [w686] -> w681
          stop <- w684 stop-if-true
          n442 = Build Array("OUI", "NON") -> (w689:bool[])
          n443 = Boolean Array To Number(Boolean array=w689) -> (number=w688:u32)
          n444 = case shown="1" w688 {
            tunnel: [FALSE TRUE w702] -> w685
            tunnel: [FALSE FALSE w702] -> w687
            frame 0, Default {
            }
            frame 1 {
            }
            frame 2 {
              w702 = TRUE
            }
          }
          n445 = local read "STOP"() -> (w683:bool)
          n446 = case shown="False" w683 {
            frame False {
              n447 = flat-sequence {
                frame #0 {
                  w694 = TRUE
                  n448 = local write "LED2"(FALSE) -> ()
                  n449 = local write "LED1"(w694) -> ()
                  n450 = local write "LED3"(w694) -> ()
                  n451 = Wait Until Next ms Multiple(millisecond multiple=1000) -> ()  [unwired: 1 out]
                }
                frame #1 {
                  w696 = FALSE
                  n452 = local write "LED2"(TRUE) -> ()
                  n453 = local write "LED1"(w696) -> ()
                  n454 = local write "LED3"(w696) -> ()
                  n455 = Wait Until Next ms Multiple(millisecond multiple=1000) -> ()  [unwired: 1 out]
                }
              }
            }
            frame True {
            }
          }
          n456 = Or(x=w683, y=w685) -> (x .or. y?=w684:bool)
          n457 = Or(x=w687, y=w683) -> (x .or. y?=w686:bool)
        }
      }
      frame #6 {
        n458 = TCP Close Connection "TCP Fermer la connexion"(connection ID=w703) -> ()  [unwired: 2 in, 2 out]
      }
    }
    n459 = Or(x="STOP", y=w1) -> (x .or. y?=w3:bool)
  }
